vi "CAEN_HVChannel.get data to modify.vi"(0 "i ref in":refnum<vi>, 3 "ms timeout (10000)":i32=10000, 5 "error in (no error)":errorcluster) -> (14 "i ref out":refnum<vi>, 16 "i attribute":T1 {"Channel Array"."TripExt"."TripExt#Multiplier" format="%#.1e"; "Channel Array"."TripInt"."TripInt#Multiplier" format="%#.1e"; "Channel Array"."IMon"."IMon#Multiplier" format="%#.1e"; "Channel Array"."VMon"."VMon#Multiplier" format="%#.1e"; "Channel Array"."SVMax"."SVMax#Multiplier" format="%#.1e"; "Channel Array"."Trip"."Trip#Multiplier" format="%#.1e"; "Channel Array"."RDWn"."RDWn#Multiplier" format="%#.1e"; "Channel Array"."RUp"."RUp#Multiplier" format="%#.1e"; "Channel Array"."I1Set"."I1Set#Multiplier" format="%#.1e"; "Channel Array"."V1Set"."V1Set#Multiplier" format="%#.1e"; "Channel Array"."I0Set"."I0Set#Multiplier" format="%#.1e"; "Channel Array"."V0Set"."V0Set#Multiplier" format="%#.1e"; "Channel Array"."Status"."Status" format="%.0b"}, 17 "timed out":bool, 19 "error out":errorcluster)   [LabVIEW 2014, in "CAEN_HVChannel.lvlib"]
doc: "Reads the attribute data of the object after the access to the data has been locked by the \"acquire\" method. If the attribute data has been locked already, this methods waits until the attribute data is unlocked or there is a timeout.\n\nThe attribute data must be unlocked using the methods \"release\" or \"set modified data\".\n\nLicense Agreement for this software:\n\nCopyright (C)\nGesellschaft für Schwerionenforschung, GSI\nPlanckstr. 1\n64291 Darmstadt\nGermany\n\nContact: D.Beck@gsi.de \n\nThis program is free software; you can redistribute it and/or modify it under the terms of the GNU General Public License as published by the Free Software Foundation; either version 2 of the license, or (at your option) any later version.\n\nThis program is distributed in the hope that it will be useful, but WITHOUT ANY WARRANTY; without even the implied warranty of MERCHANTABILITY or FITNESS FOR A PARTICULAR PURPOSE. See the GNU General License for more details (http://www.gnu.org).\n\nGesellschaft für Schwerionenforschung, GSI\nPlanckstr. 1, 64291 Darmstadt, Germany\nFor all questions and ideas contact: M.Richter@gsi.de, H.Brand@gsi.de or D.Beck@gsi.de.\nLast update: 17-JUN-2004"
uses:
  CAEN_HVChannel.lvlib
  CAEN_HVChannel.i attribute.ctl
  CS_Core/CSObj/CSObj.lvlib
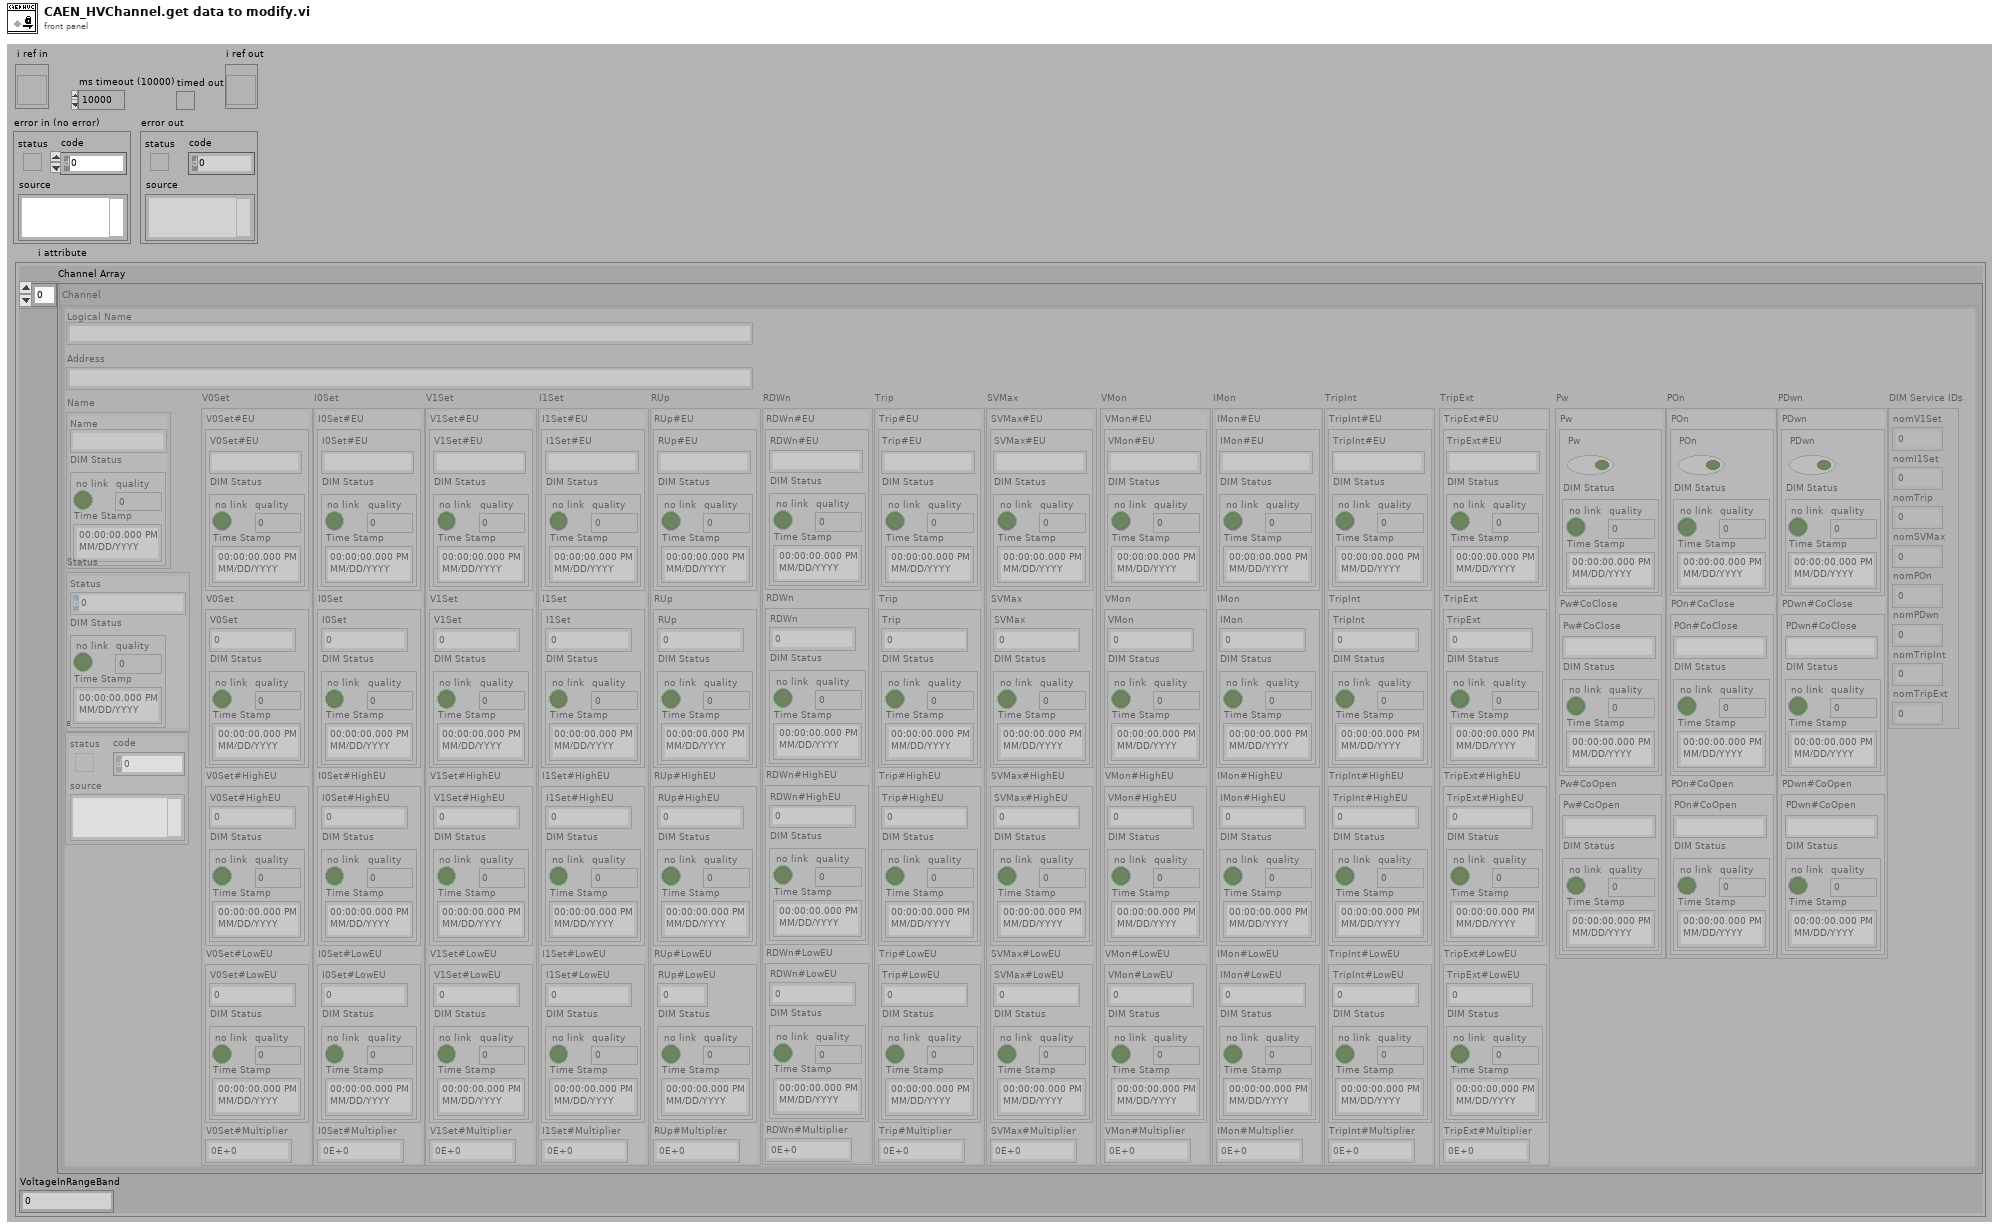
[diagram p1: front panel]
types:
  T1 = typedef "CAEN_HVChannel.lvlib/CAEN_HVChannel.i attribute.ctl" = cluster{"Channel Array":cluster{"Logical Name":string, "Address":string, "error in (no error)":errorcluster, "Name":cluster{"Name":string, "DIM Status":cluster{"no link":bool, "quality":i32, "Time Stamp":timestamp}}, "Status":cluster{"Status":i16, "DIM Status":cluster{"no link":bool, "quality":i32, "Time Stamp":timestamp}}, "V0Set":cluster{"V0Set#EU":cluster{"V0Set#EU":string, "DIM Status":cluster{"no link":bool, "quality":i32, "Time Stamp":timestamp}}, "V0Set":cluster{"V0Set":dbl, "DIM Status":cluster{"no link":bool, "quality":i32, "Time Stamp":timestamp}}, "V0Set#HighEU":cluster{"V0Set#HighEU":dbl, "DIM Status":cluster{"no link":bool, "quality":i32, "Time Stamp":timestamp}}, "V0Set#LowEU":cluster{"V0Set#LowEU":dbl, "DIM Status":cluster{"no link":bool, "quality":i32, "Time Stamp":timestamp}}, "V0Set#Multiplier":dbl}, "I0Set":cluster{"I0Set#EU":cluster{"I0Set#EU":string, "DIM Status":cluster{"no link":bool, "quality":i32, "Time Stamp":timestamp}}, "I0Set":cluster{"I0Set":dbl, "DIM Status":cluster{"no link":bool, "quality":i32, "Time Stamp":timestamp}}, "I0Set#HighEU":cluster{"I0Set#HighEU":dbl, "DIM Status":cluster{"no link":bool, "quality":i32, "Time Stamp":timestamp}}, "I0Set#LowEU":cluster{"I0Set#LowEU":dbl, "DIM Status":cluster{"no link":bool, "quality":i32, "Time Stamp":timestamp}}, "I0Set#Multiplier":dbl}, "V1Set":cluster{"V1Set#EU":cluster{"V1Set#EU":string, "DIM Status":cluster{"no link":bool, "quality":i32, "Time Stamp":timestamp}}, "V1Set":cluster{"V1Set":dbl, "DIM Status":cluster{"no link":bool, "quality":i32, "Time Stamp":timestamp}}, "V1Set#HighEU":cluster{"V1Set#HighEU":dbl, "DIM Status":cluster{"no link":bool, "quality":i32, "Time Stamp":timestamp}}, "V1Set#LowEU":cluster{"V1Set#LowEU":dbl, "DIM Status":cluster{"no link":bool, "quality":i32, "Time Stamp":timestamp}}, "V1Set#Multiplier":dbl}, "I1Set":cluster{"I1Set#EU":cluster{"I1Set#EU":string, "DIM Status":cluster{"no link":bool, "quality":i32, "Time Stamp":timestamp}}, "I1Set":cluster{"I1Set":dbl, "DIM Status":cluster{"no link":bool, "quality":i32, "Time Stamp":timestamp}}, "I1Set#HighEU":cluster{"I1Set#HighEU":dbl, "DIM Status":cluster{"no link":bool, "quality":i32, "Time Stamp":timestamp}}, "I1Set#LowEU":cluster{"I1Set#LowEU":dbl, "DIM Status":cluster{"no link":bool, "quality":i32, "Time Stamp":timestamp}}, "I1Set#Multiplier":dbl}, "RUp":cluster{"RUp#EU":cluster{"RUp#EU":string, "DIM Status":cluster{"no link":bool, "quality":i32, "Time Stamp":timestamp}}, "RUp":cluster{"RUp":dbl, "DIM Status":cluster{"no link":bool, "quality":i32, "Time Stamp":timestamp}}, "RUp#HighEU":cluster{"RUp#HighEU":dbl, "DIM Status":cluster{"no link":bool, "quality":i32, "Time Stamp":timestamp}}, "RUp#LowEU":cluster{"RUp#LowEU":dbl, "DIM Status":cluster{"no link":bool, "quality":i32, "Time Stamp":timestamp}}, "RUp#Multiplier":dbl}, "RDWn":cluster{"RDWn#EU":cluster{"RDWn#EU":string, "DIM Status":cluster{"no link":bool, "quality":i32, "Time Stamp":timestamp}}, "RDWn":cluster{"RDWn":dbl, "DIM Status":cluster{"no link":bool, "quality":i32, "Time Stamp":timestamp}}, "RDWn#HighEU":cluster{"RDWn#HighEU":dbl, "DIM Status":cluster{"no link":bool, "quality":i32, "Time Stamp":timestamp}}, "RDWn#LowEU":cluster{"RDWn#LowEU":dbl, "DIM Status":cluster{"no link":bool, "quality":i32, "Time Stamp":timestamp}}, "RDWn#Multiplier":dbl}, "Trip":cluster{"Trip#EU":cluster{"Trip#EU":string, "DIM Status":cluster{"no link":bool, "quality":i32, "Time Stamp":timestamp}}, "Trip":cluster{"Trip":dbl, "DIM Status":cluster{"no link":bool, "quality":i32, "Time Stamp":timestamp}}, "Trip#HighEU":cluster{"Trip#HighEU":dbl, "DIM Status":cluster{"no link":bool, "quality":i32, "Time Stamp":timestamp}}, "Trip#LowEU":cluster{"Trip#LowEU":dbl, "DIM Status":cluster{"no link":bool, "quality":i32, "Time Stamp":timestamp}}, "Trip#Multiplier":dbl}, "SVMax":cluster{"SVMax#EU":cluster{"SVMax#EU":string, "DIM Status":cluster{"no link":bool, "quality":i32, "Time Stamp":timestamp}}, "SVMax":cluster{"SVMax":dbl, "DIM Status":cluster{"no link":bool, "quality":i32, "Time Stamp":timestamp}}, "SVMax#HighEU":cluster{"SVMax#HighEU":dbl, "DIM Status":cluster{"no link":bool, "quality":i32, "Time Stamp":timestamp}}, "SVMax#LowEU":cluster{"SVMax#LowEU":dbl, "DIM Status":cluster{"no link":bool, "quality":i32, "Time Stamp":timestamp}}, "SVMax#Multiplier":dbl}, "VMon":cluster{"VMon#EU":cluster{"VMon#EU":string, "DIM Status":cluster{"no link":bool, "quality":i32, "Time Stamp":timestamp}}, "VMon":cluster{"VMon":dbl, "DIM Status":cluster{"no link":bool, "quality":i32, "Time Stamp":timestamp}}, "VMon#HighEU":cluster{"VMon#HighEU":dbl, "DIM Status":cluster{"no link":bool, "quality":i32, "Time Stamp":timestamp}}, "VMon#LowEU":cluster{"VMon#LowEU":dbl, "DIM Status":cluster{"no link":bool, "quality":i32, "Time Stamp":timestamp}}, "VMon#Multiplier":dbl}, "IMon":cluster{"IMon#EU":cluster{"IMon#EU":string, "DIM Status":cluster{"no link":bool, "quality":i32, "Time Stamp":timestamp}}, "IMon":cluster{"IMon":dbl, "DIM Status":cluster{"no link":bool, "quality":i32, "Time Stamp":timestamp}}, "IMon#HighEU":cluster{"IMon#HighEU":dbl, "DIM Status":cluster{"no link":bool, "quality":i32, "Time Stamp":timestamp}}, "IMon#LowEU":cluster{"IMon#LowEU":dbl, "DIM Status":cluster{"no link":bool, "quality":i32, "Time Stamp":timestamp}}, "IMon#Multiplier":dbl}, "TripInt":cluster{"TripInt#EU":cluster{"TripInt#EU":string, "DIM Status":cluster{"no link":bool, "quality":i32, "Time Stamp":timestamp}}, "TripInt":cluster{"TripInt":dbl, "DIM Status":cluster{"no link":bool, "quality":i32, "Time Stamp":timestamp}}, "TripInt#HighEU":cluster{"TripInt#HighEU":dbl, "DIM Status":cluster{"no link":bool, "quality":i32, "Time Stamp":timestamp}}, "TripInt#LowEU":cluster{"TripInt#LowEU":dbl, "DIM Status":cluster{"no link":bool, "quality":i32, "Time Stamp":timestamp}}, "TripInt#Multiplier":dbl}, "TripExt":cluster{"TripExt#EU":cluster{"TripExt#EU":string, "DIM Status":cluster{"no link":bool, "quality":i32, "Time Stamp":timestamp}}, "TripExt":cluster{"TripExt":dbl, "DIM Status":cluster{"no link":bool, "quality":i32, "Time Stamp":timestamp}}, "TripExt#HighEU":cluster{"TripExt#HighEU":dbl, "DIM Status":cluster{"no link":bool, "quality":i32, "Time Stamp":timestamp}}, "TripExt#LowEU":cluster{"TripExt#LowEU":dbl, "DIM Status":cluster{"no link":bool, "quality":i32, "Time Stamp":timestamp}}, "TripExt#Multiplier":dbl}, "Pw":cluster{"Pw":cluster{"Pw":bool, "DIM Status":cluster{"no link":bool, "quality":i32, "Time Stamp":timestamp}}, "Pw#CoClose":cluster{"Pw#CoClose":string, "DIM Status":cluster{"no link":bool, "quality":i32, "Time Stamp":timestamp}}, "Pw#CoOpen":cluster{"Pw#CoOpen":string, "DIM Status":cluster{"no link":bool, "quality":i32, "Time Stamp":timestamp}}}, "POn":cluster{"POn":cluster{"POn":bool, "DIM Status":cluster{"no link":bool, "quality":i32, "Time Stamp":timestamp}}, "POn#CoClose":cluster{"POn#CoClose":string, "DIM Status":cluster{"no link":bool, "quality":i32, "Time Stamp":timestamp}}, "POn#CoOpen":cluster{"POn#CoOpen":string, "DIM Status":cluster{"no link":bool, "quality":i32, "Time Stamp":timestamp}}}, "PDwn":cluster{"PDwn":cluster{"PDwn":bool, "DIM Status":cluster{"no link":bool, "quality":i32, "Time Stamp":timestamp}}, "PDwn#CoClose":cluster{"PDwn#CoClose":string, "DIM Status":cluster{"no link":bool, "quality":i32, "Time Stamp":timestamp}}, "PDwn#CoOpen":cluster{"PDwn#CoOpen":string, "DIM Status":cluster{"no link":bool, "quality":i32, "Time Stamp":timestamp}}}, "DIM Service IDs":cluster{"nomV1Set":i32, "nomI1Set":i32, "nomTrip":i32, "nomSVMax":i32, "nomPOn":i32, "nomPDwn":i32, "nomTripInt":i32, "nomTripExt":i32}}[], "VoltageInRangeBand":dbl}
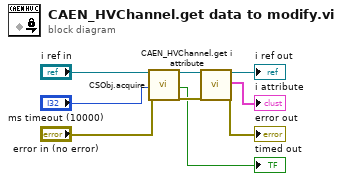
[diagram p0: block diagram]
diagram:
  n1 = call "CSObj.acquire.vi"("i ref in"="i ref in", "ms timeout (10000)"="ms timeout (10000)", "error in (no error)"="error in (no error)") -> ("i ref out"=w8:refnum<vi>, "timed out"=→"timed out":bool, "error out"=w5:errorcluster)  [unwired: 14 in]
  n2 = call "CAEN_HVChannel.get i attribute.vi"("i ref in"=w8, "error in (no error)"=w5) -> ("i ref out"=→"i ref out":refnum<vi>, "i attribute"=→"i attribute":T1, "error out"=→"error out":errorcluster)  [unwired: 15 in]
